vi "tdsstop.vi"(2 "Error In (No Error)":errorcluster, 3 "VISA Port In":refnum<visa-resource-name>) -> (0 "Error Out":errorcluster, 1 "VISA Port Out":refnum<visa-resource-name>)   [LabVIEW 2011]
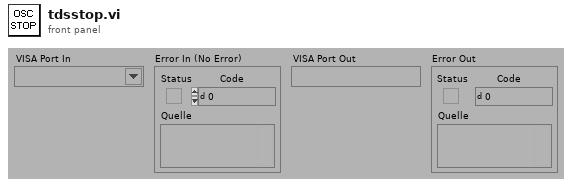
[diagram p1: front panel]
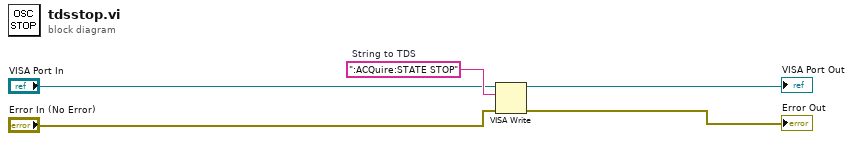
[diagram p0: block diagram]
diagram:
  w5 = ":ACQuire:STATE STOP"  # String to TDS
  n1 = VISA Write(VISA resource name="VISA Port In", write buffer=w5, error in (no error)="Error In (No Error)") -> (VISA resource name out=→"VISA Port Out":refnum<visa-resource-name>, error out=→"Error Out":errorcluster)  [unwired: 1 out]
